vi "Example - Fetch a Table.vi"() -> ()   [LabVIEW 2013]
doc: "This example opens a connection to a database specified by the Connection string (replace the DNS name with your database) and retrieves all the rows and columns from the table \"Table1\" (replace the SQL string with your own SQL query)."
panel:
  out "error out":errorcluster
  out "SQL Results":string[][](table)
  in  "Command Text":string="SELECT * FROM myTable WHERE Age < 30;"
  in  "ConnectionString":string="DSN=myDB;"
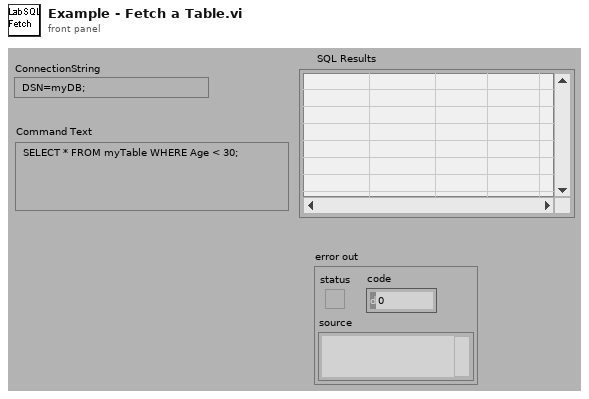
[diagram p1: front panel]
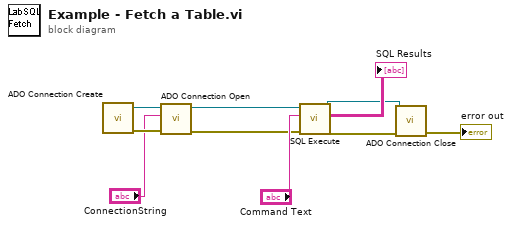
[diagram p0: block diagram]
diagram:
  n1 = call "ADO Connection Create.vi"() -> ("error out"=w9:errorcluster, "ADODB._Connection Out"=w10:refnum<k7>)  [unwired: 10 in]
  n2 = call "ADO Connection Open.vi"("error in (no error)"=w9, "ConnectionString"="ConnectionString", "ADODB._Connection In"=w10) -> ("error out"=w5:errorcluster, "ADODB._Connection Out"=w7:refnum<k7>)  [unwired: 7 in]
  n3 = call "SQL Execute.vi"("error in (no error)"=w5, "Command Text"="Command Text", "ADODB._Connection In"=w7) -> ("error out"=w3:errorcluster, "Data"=→"SQL Results":string[][], "ADODB._Connection Out"=w2:refnum<k7>)  [unwired: 5 in, 1 out]
  n4 = call "ADO Connection Close.vi"("error in (no error)"=w3, "ADODB._Connection In"=w2) -> ("error out"=→"error out":errorcluster)  [unwired: 8 in, 1 out]
